vi "Chicharronera.vi"() -> ()   [LabVIEW 2018]
panel:
  in  "stop":bool
  out "X2":dbl
  out "X1":dbl
  in  "c":dbl
  in  "b":dbl
  in  "a":dbl
  # "La Chicharronera"
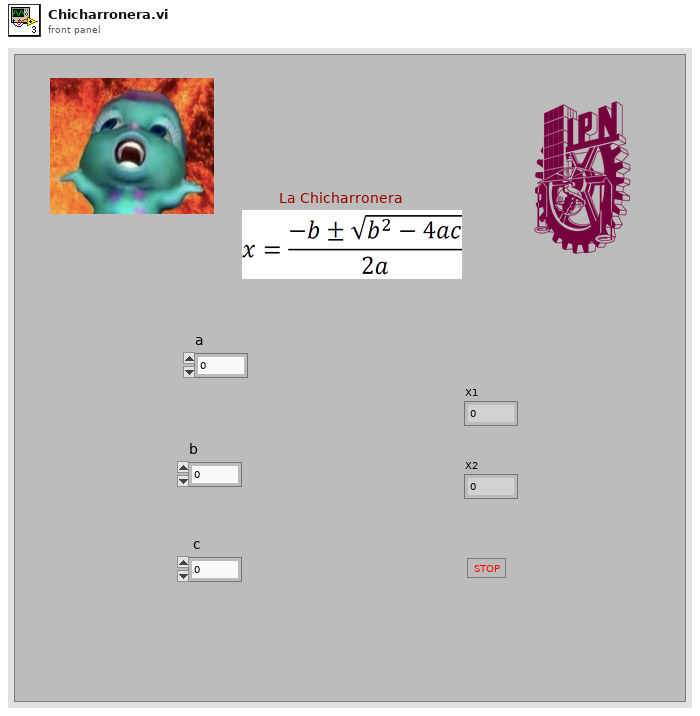
[diagram p1: front panel]
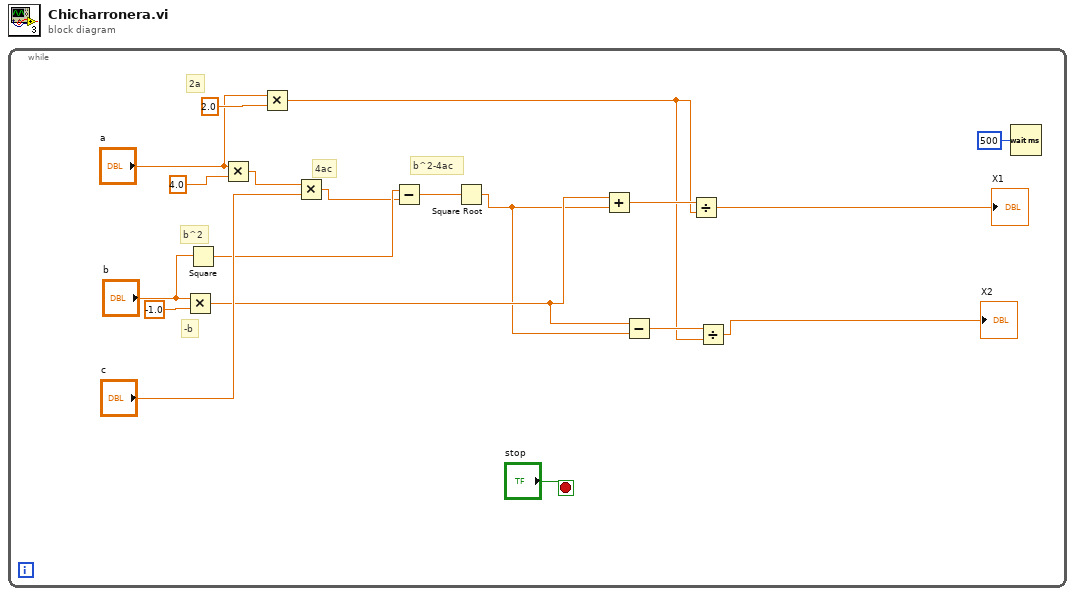
[diagram p0: block diagram]
diagram:
  n1 = while {
    stop <- "stop" stop-if-true
    # "2a"
    # "-b"
    # "b^2-4ac"
    # "b^2"
    # "4ac"
    n2 = Multiply(x="b", y=-1.0) -> (x*y=w5:dbl)
    n3 = Square(x="b") -> (x^2=w12:dbl)
    n4 = Multiply(x="a", y=4.0) -> (x*y=w15:dbl)
    n5 = Multiply(x="a", y=2.0) -> (x*y=w2:dbl)
    n6 = Multiply(x=w15, y="c") -> (x*y=w11:dbl)
    n7 = Subtract(x=w12, y=w11) -> (x-y=w10:dbl)
    n8 = Square Root(x=w10) -> (sqrt(x)=w4:dbl)
    n9 = Add(x=w5, y=w4) -> (x+y=w7:dbl)
    n10 = Subtract(x=w5, y=w4) -> (x-y=w3:dbl)
    n11 = Divide(x=w7, y=w2) -> (x/y=→"X1":dbl)
    n12 = Divide(x=w3, y=w2) -> (x/y=→"X2":dbl)
    n13 = Wait (ms)(milliseconds to wait=u32 500) -> ()  [unwired: 1 out]
  }
